vi "Test Main.vi"   [LabVIEW 2020, in "VolatusScratch.lvlib"]
uses:
  VolatusScratch.lvlib
  Volatus/Volatus Core/Volatus Core.lvclass
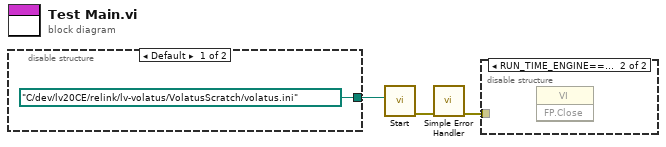
[diagram p0: block diagram]
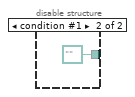
[diagram p3: hidden frame]
diagram:
  n1 = disable-structure shown="Default" {
    disable-tunnel: [path "C:/dev/lv20CE/relink/lv-volatus/VolatusScratch/volatus.ini" ("INI Path (Default)") path "" ("INI Path (Default)")] -> w3
    frame condition #0 (active) {
    }
    frame condition #1 {
    }
  }
  n2 = call "Start.vi"("INI Path (Default)"=w3) -> ("error out"=w1:errorcluster)  [unwired: 9 in, 1 out]
  n3 = call <vilib>:"Simple Error Handler.vi"("error in (no error)"=w1) -> ("error out"=w2:errorcluster)  [unwired: 4 in, 4 out]
  n4 = disable-structure shown="RUN_TIME_ENGINE==True" {
    disable-tunnel: w2 -> [_ _]
    frame condition #0 (active) {
    }
    frame condition #1 {
      n5 = invoke class="VI" method="FP.Close"() -> ()  [unwired: 3 in, 3 out]
    }
  }
